vi "Receive User Menu Selection Msg.vi"(8 "error in (no error)":errorcluster, 10 "UserMenuSelectionMsg":refnum<class "UserMenuSelectionMsg.lvclass">, 11 "ActorAutoRegistrationView In":refnum<class "ActorAutoRegistrationView.lvclass">) -> (0 "error out":errorcluster, 3 "ActorAutoRegistrationView Out":refnum<class "ActorAutoRegistrationView.lvclass">)   [LabVIEW 2015, in "TestViewables.lvlib" / "ActorAutoRegistrationView.lvclass"]
doc: "<License>\nCopyright © 2017 Composed Systems, LLC | All rights reserved\nwww.composed.io\n\nAuthor: Ethan Stern <ethan.stern@composed.io>\n\nThis software is provided \"AS IS\" WITHOUT WARRANTIES, either express or implied, AND IS FOR EDUCATIONAL PURPOSES ONLY.\n</License>"
uses:
  ActorAutoRegistrationView.lvclass
  Framework/AutoRegistration/ActorAutoRegistration Messages/UserMenuSelectionMsg/UserMenuSelectionMsg.lvclass
  DialogBox/OneButtonDialogBox/OneButtonDialogBox.lvclass
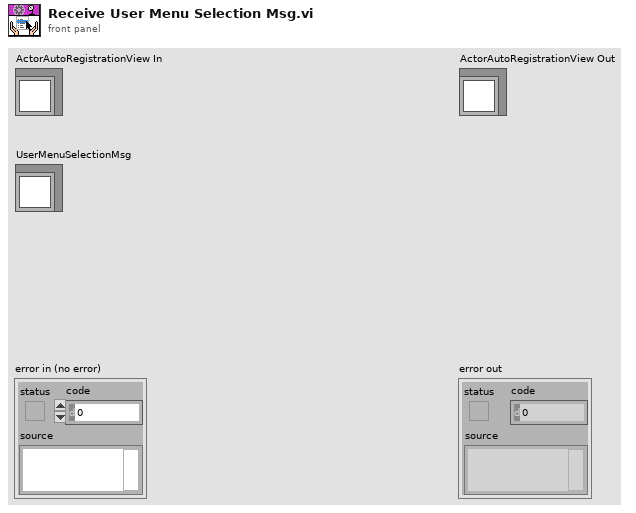
[diagram p1: front panel]
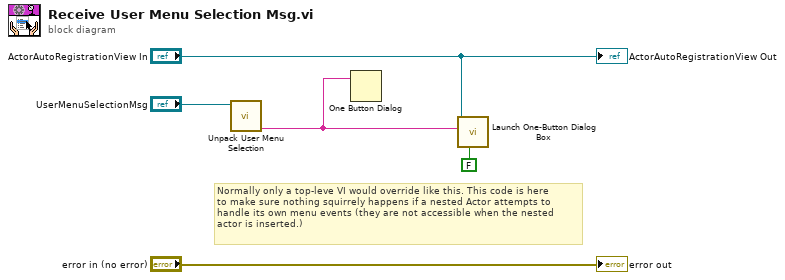
[diagram p0: block diagram]
diagram:
  # "Normally only a top-leve VI would override like this. This code is here\nto make sure nothing squirrely happens if a nested Actor attempts to\nhandle its own menu events (they are not accessible when the nested\nactor is inserted.)"
  n1 = call-dynamic "Unpack User Menu Selection.vi"("UserMenuSelectionMsg In"="UserMenuSelectionMsg") -> ("Item Path"=w1:string)  [unwired: 7 in, 3 out]
  n2 = One Button Dialog(message=w1) -> ()  [unwired: 1 in, 1 out]
  n3 = call "Launch One-Button Dialog Box.vi"("Modal? (T)"=FALSE, "Message Text"=w1, "Dialog Launcher"="ActorAutoRegistrationView In") -> ()  [unwired: 8 in, 1 out]
  "error out" <- "error in (no error)"
  "ActorAutoRegistrationView Out" <- "ActorAutoRegistrationView In"
